vi "Timer_MacroGen.vi"(7 "Timer Command":T1, 8 "Error In":errorcluster, 11 "Set Time (ms)":dbl) -> (0 "Error Out":errorcluster, 1 "Remaining Time (ms)":dbl, 2 "Elapsed Time (ms)":dbl, 3 "Complete?":bool)   [LabVIEW 2012]
doc: "This FGV implements a timer.\nFunctionality is a follows:\n1. START the timer first (using the command enum and specifying the timing duration.\n2. Calling the VI with 'RUN' returns the elapsed time, remaining time and indication weather complete\n3. A PAUSE functionality is also provided which allows you to suspend the timing till RUN is called again"
uses:
  Timer_MacroGen_Commands.ctl
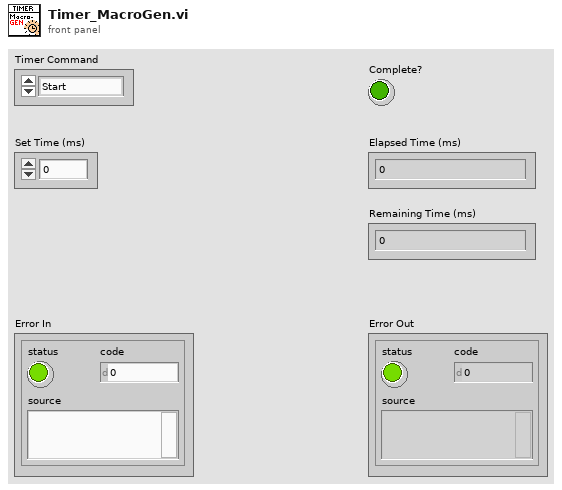
[diagram p1: front panel]
types:
  T1 = typedef "Timer_MacroGen_Commands.ctl" = enum16{"Start", "Pause", "Run"}
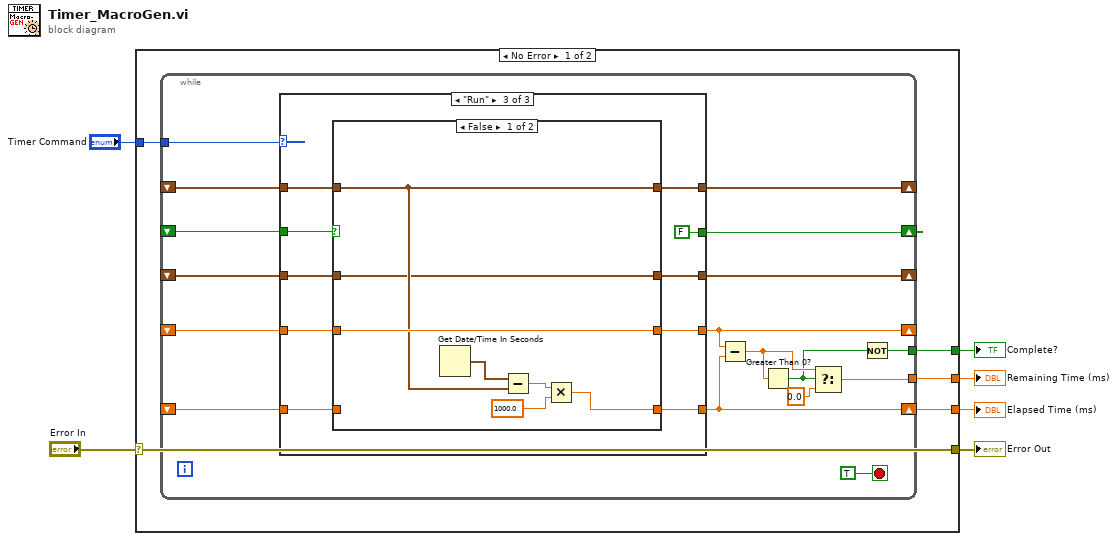
[diagram p0: block diagram]
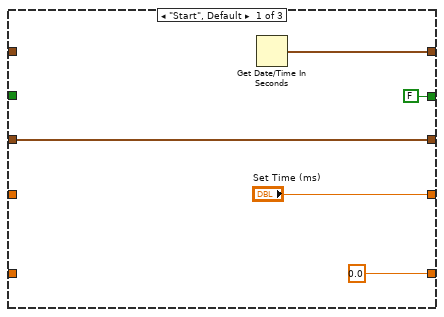
[diagram p2: hidden frame]
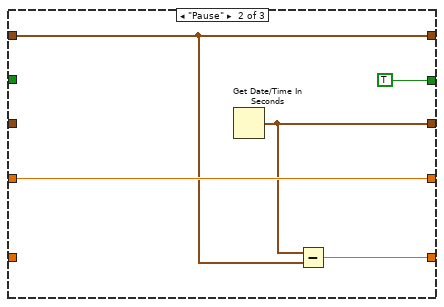
[diagram p3: hidden frame]
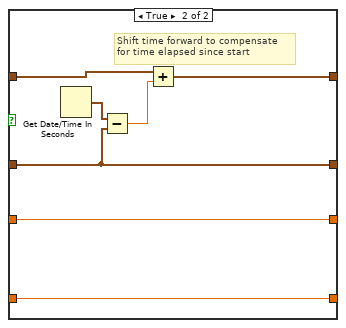
[diagram p4: hidden frame]
diagram:
  n1 = case shown="No Error" "Error In" {
    selector: "Error In" -> [w10 w63]
    tunnel: [w10 w63] -> w5
    tunnel: "Timer Command" -> [w11 _]
    tunnel: [w9 _] -> w3
    tunnel: [w8 _] -> w2
    tunnel: [w7 _] -> w1
    frame No Error {
      n2 = while {
        tunnel: w11 -> [w27]
        shift-right: [w18] -> _
        shift-left: _ -> [w22]
        shift-right: [w26] -> _
        shift-left: _ -> [w25]
        shift-right: [w24] -> _
        shift-left: _ -> [w23]
        shift-right: [w21] -> _
        shift-left: _ -> [w20]
        shift-right: [w17] -> w9
        shift-left: _ -> [w19]
        tunnel: [w15] -> w8
        tunnel: [w13] -> w7
        stop <- TRUE stop-if-true
        n3 = case shown="\"Run\"" w27 {
          tunnel: ["Set Time (ms)" w37 w39] -> w18
          tunnel: [w32 w35 w43] -> w26
          tunnel: w25 -> [_ w35 w46]
          tunnel: [FALSE TRUE FALSE] -> w24
          tunnel: w23 -> [_ _ w47]
          tunnel: w22 -> [_ w37 w44]
          tunnel: [w30 w36 w40] -> w21
          tunnel: w20 -> [w30 _ w45]
          tunnel: [0.0 w34 w42] -> w17
          tunnel: w19 -> [_ _ w41]
          frame "Start", Default {
            n4 = Get Date/Time In Seconds() -> (seconds since 1Jan1904=w32:timestamp)
          }
          frame "Pause" {
            n5 = Get Date/Time In Seconds() -> (seconds since 1Jan1904=w36:timestamp)
            n6 = Subtract(x=w36, y=w35) -> (x-y=w34:dbl)
          }
          frame "Run" {
            n7 = case shown="False" w47 {
              tunnel: w46 -> [w53 w59]
              tunnel: w45 -> [w52 w56]
              tunnel: w44 -> [w54 w61]
              tunnel: [w53 w57] -> w43
              tunnel: [w49 w62] -> w42
              tunnel: w41 -> [_ w62]
              tunnel: [w52 w56] -> w40
              tunnel: [w54 w61] -> w39
              frame False {
                n8 = Get Date/Time In Seconds() -> (seconds since 1Jan1904=w55:timestamp)
                n9 = Subtract(x=w55, y=w53) -> (x-y=w51:dbl)
                n10 = Multiply(x=w51, y=1000.0) -> (x*y=w49:dbl)
              }
              frame True {
                # "Shift time forward to compensate\nfor time elapsed since start"
                n11 = Get Date/Time In Seconds() -> (seconds since 1Jan1904=w60:timestamp)
                n12 = Subtract(x=w60, y=w56) -> (x-y=w58:dbl)
                n13 = Add(x=w59, y=w58) -> (x+y=w57:timestamp)
              }
            }
          }
        }
        n14 = Subtract(x=w18, y=w17) -> (x-y=w14:dbl)
        n15 = Greater Than 0?(x=w14) -> (x > 0?=w12:bool)
        n16 = Select(t=w14, s=w12, f=0.0) -> (s? t:f=w15:dbl)
        n17 = Not(x=w12) -> (.not. x?=w13:bool)
      }
    }
    frame Error {
    }
  }
  "Error Out" <- w5
  "Complete?" <- w1
  "Remaining Time (ms)" <- w2
  "Elapsed Time (ms)" <- w3
